vi "Main.vi"() -> ()   [LabVIEW 2018]
uses:
  Initialize/CreateQueue/AllDataQueue.ctl
  Initialize/CreateQueue/SocketQueue.ctl
  Initialize/CreateQueue/LogDataQueue.ctl
  Initialize/CreateQueue/ProDataQueue.ctl
  ProData/SettingData.ctl
  socket/socket.ctl
  Initialize/Setting/DA.ctl
  Initialize/Setting/AD.ctl
  ProData/prodatascan.ctl
  Support/Data.ctl
  <vilib>/DAQmx/read.llb/DAQmx Read (Analog Wfm 1Chan NSamp).vi
  <vilib>/DAQmx/write.llb/DAQmx Write (Analog DBL 1Chan 1Samp).vi
  <vilib>/DAQmx/create/channels.llb/DAQmx Create Channel (AI-Voltage-Basic).vi
  <vilib>/DAQmx/configure/timing.llb/DAQmx Timing (Sample Clock).vi
  <vilib>/DAQmx/miscellaneous.llb/DAQmx Fill In Error Info.vi
  <vilib>/DAQmx/create/channels.llb/DAQmx Create Channel (AO-Voltage-Basic).vi
panel:
  in  "选项卡控件":enum32{"Setting", "Chart"}(tab)
  in  "port":dbl=10003.0
  in  "timeout":i16=-1
  in  "标准差倍数":dbl=5.0
  in  "normal":string="1"
  in  "每通道采样率":u16=60
  in  "电压最大值":u16=5
  in  "电压最小值":i16=-5
  in  "采样率":u16=60000
  in  "接线方式":i32(ring)=10106 items=["默认"=-1, "RSE"=10083, "NRSE"=10078, "差分"=10106, "伪差分"=12529]
  in  "采样模式":i32(ring)=10123 items=["有限采样"=10178, "连续采样"=10123, "硬件定时单点"=12522]
  in  "DA电压最大值":dbl=10.0
  in  "DA电压最小值":dbl=-10.0
  in  "选择通道AD":tag="USB_6211_C34SF/ai1"
  in  "选择通道DA":tag="USB_6211_C34SF/ao1"
  in  "地址":string="8.131.237.84"
  out "选择通道AD  2":tag="USB_6211_2/ai1"
  out "连接状态":string="连接成功"
  in  "adjust":dbl=0.1
  out "波形图表":i32(graph)
  out "nvpai":dbl
  out "max":dbl
  out "min":dbl
  in  "等待时间（毫秒）":u32=20
  out "ADchart":dbl(graph)
  out "DAchart":dbl(graph)
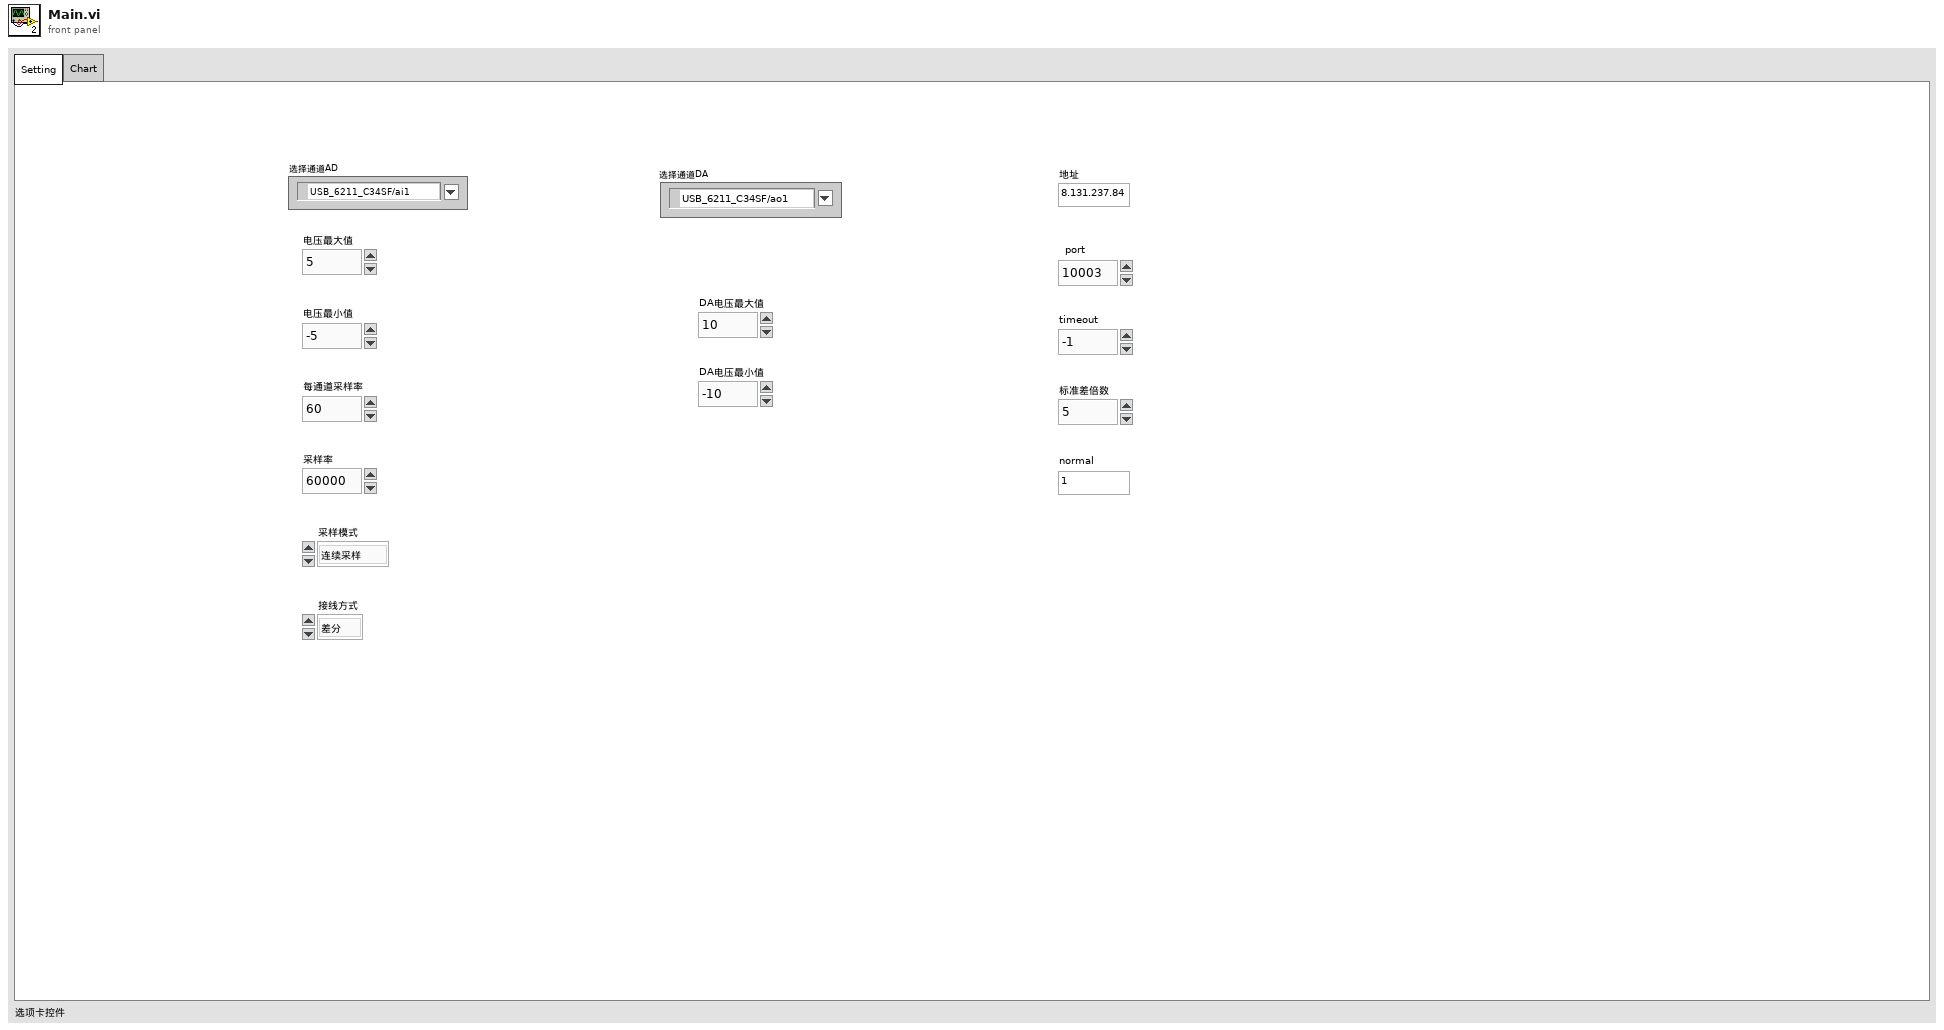
[diagram p1: front panel]
types:
  T1 = typedef "socket.ctl" = cluster{"端口":u16, "timeout":u16, "标准差倍数":dbl, "address":string, "abnormal":string}
  T2 = typedef "DA.ctl" = cluster{"电压最大值":dbl, " 电压最小值":dbl, "选择通道DA ":tag}
  T3 = typedef "AD.ctl" = cluster{"电压最大值":u16, " 电压最小值":i16, " 采样率":u16, "每通道采样率":u16, "采样模式":i32, "接线方式":i32, "source":tag, "选择通道AD ":tag}
  T4 = typedef "Data.ctl" = cluster{"SynQueue":cluster{"SocketQueue":T5, "LogQueue":T6, " DA":refnum<queue>, "ProQueue":T7}, "Error":cluster{"错误输出 2":errorcluster}, "SettingData":T8}
  T5 = typedef "SocketQueue.ctl" = cluster{"ADSTDqueue ":refnum<queue>, "SocketADExceptionqueue":refnum<queue>, "  SocketAD":refnum<queue>}
  T6 = typedef "LogDataQueue.ctl" = cluster{"RunningADqueue":refnum<queue>, "Compensatequeue":refnum<queue>, " RunningDAqueue":refnum<queue>, " RunMin":refnum<queue>}
  T7 = typedef "ProDataQueue.ctl" = cluster{"buffer ":refnum<queue>, " StimeADqueue":refnum<queue>, "  MtimeADqueue":refnum<queue>}
  T8 = typedef "SettingData.ctl" = cluster{"socket":T1, "DA":T2, "AD":T3, "prodatascan":T9}
  T9 = typedef "prodatascan.ctl" = cluster{"max":dbl, "min":dbl, " nvpai":dbl, "初始化数组":dbl[]}
  T10 = typedef "AllDataQueue.ctl" = cluster{"SocketQueue":T5, "LogQueue":T6, " DA":refnum<queue>, "ProQueue":T7}
  T11 = cluster{"max":dbl, "min":dbl, " nvpai":dbl, "初始化数组":dbl[]}
  T12 = cluster{"SocketQueue":T5, "LogQueue":T6, " DA":refnum<queue>, "ProQueue":T7}
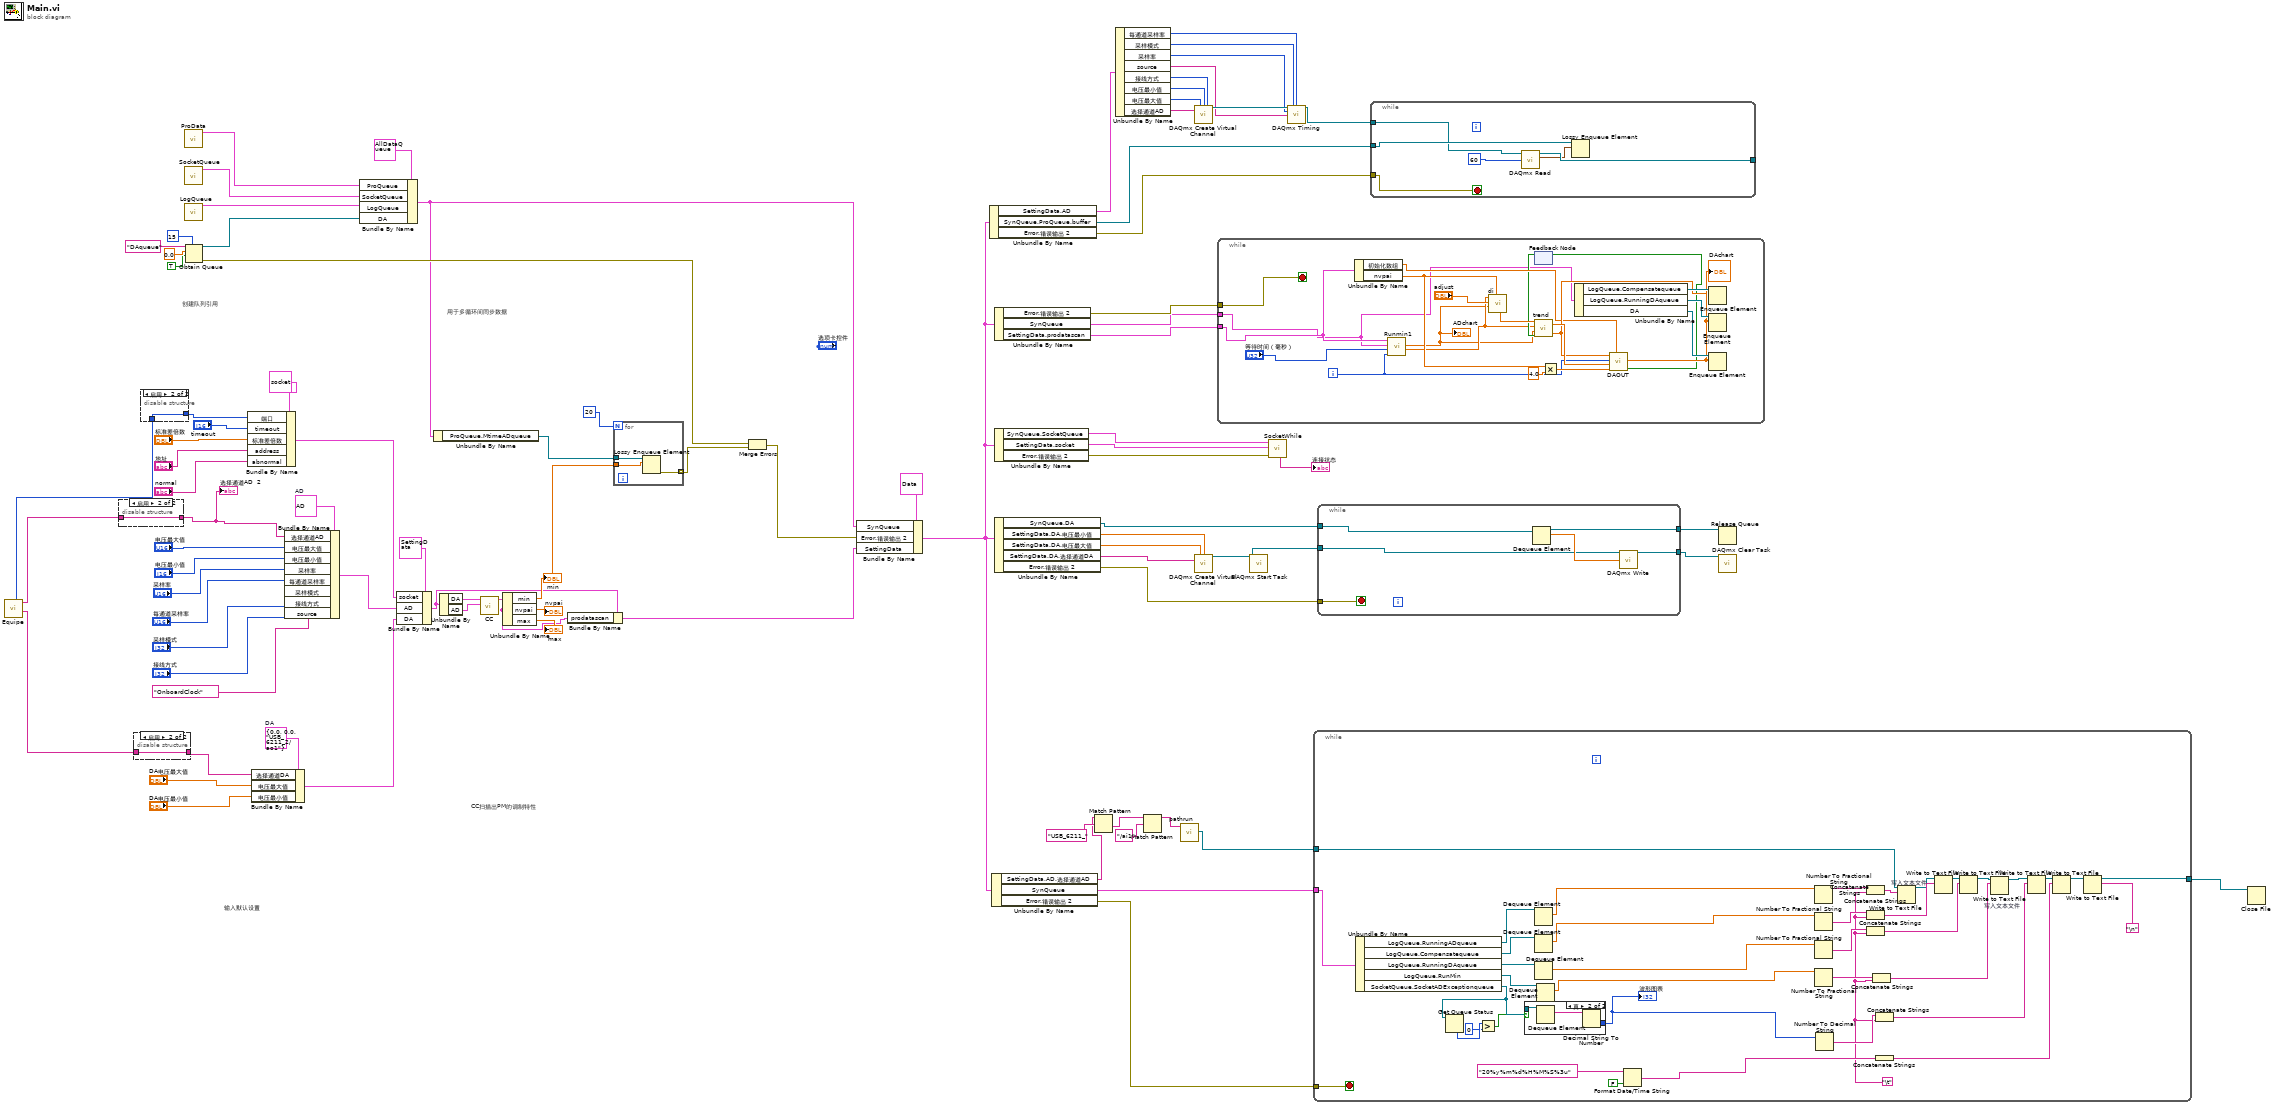
[diagram p0: block diagram]
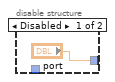
[diagram p2: hidden frame]
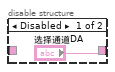
[diagram p3: hidden frame]
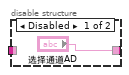
[diagram p4: hidden frame]
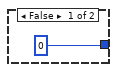
[diagram p5: hidden frame]
diagram:
  w20 = T2 {"电压最大值"=0.0, " 电压最小值"=0.0, "选择通道DA "="USB_6211_2/ao1"}  # DA
  w21 = T3 {"电压最大值"=10013, " 电压最小值"=10013, " 采样率"=10013, "每通道采样率"=10013, "采样模式"=10123, "接线方式"=10106, "source"="OnboardClock", "选择通道AD "="USB_6211_2/ai1"}  # AD
  # "CC扫描出PM的调制特性"
  # "输入默认设置"
  # "用于多循环间同步数据"
  # "创建队列引用"
  n1 = call "Equipe.vi"() -> ("DA"=w4:string, "AD"=w5:string, "port"=w3:i32)  [unwired: 8 in, 1 out]
  n2 = disable-structure shown="启用" {
    disable-tunnel: ["选择通道AD" w91] -> w6
    disable-tunnel: w5 -> [_ w91]
    frame Disabled {
    }
    frame Enabled {
    }
  }
  "选择通道AD  2" <- w6
  n3 = disable-structure shown="启用" {
    disable-tunnel: ["选择通道DA" w93] -> w67
    disable-tunnel: w4 -> [_ w93]
    frame Disabled {
    }
    frame Enabled {
    }
  }
  n4 = disable-structure shown="启用" {
    disable-tunnel: ["port" w95] -> w1
    disable-tunnel: w3 -> [_ w95]
    frame Disabled {
    }
    frame Enabled {
    }
  }
  n5 = call "ProData.vi"() -> ("ProDataQueue"=w81:T7)  [unwired: 11 in]
  n6 = call "SocketQueue.vi"() -> ("SocketQueue"=w83:T5)  [unwired: 11 in]
  n7 = call "LogQueue.vi"() -> ("LogQueue"=w82:T6)  [unwired: 11 in]
  n8 = Obtain Queue(max queue size (-1, unlimited)=15 ("队列最大值（-1，无限）"), name (unnamed)="DAqueue" ("名称（未命名）"), element data type=0.0, create if not found? (T)=TRUE ("如未找到则创建？(T)")) -> (queue out=w84:refnum<queue>, error out=w60:errorcluster)  [unwired: 1 in, 1 out]
  n9 = Bundle By Name(cluster=T1 {"端口"=10013, "timeout"=10013, "标准差倍数"=0.0, "address"="{\"ad\":1}", "abnormal"="{\"ad\":0}"} ("socket"), "端口"=w1, "timeout"="timeout", "标准差倍数"="标准差倍数", "address"="地址", "abnormal"="normal") -> (w71:T1)
  n10 = Bundle By Name(cluster=w20, "选择通道DA"=w67, "电压最大值"="DA电压最大值", "电压最小值"="DA电压最小值") -> (w66:T2)
  n11 = Bundle By Name(cluster=w21, "选择通道AD"=w6, "电压最大值"="电压最大值", "电压最小值"="电压最小值", "采样率"="采样率", "每通道采样率"="每通道采样率", "采样模式"="采样模式", "接线方式"="接线方式", "source"=tag "OnboardClock") -> (w65:T3)
  n12 = Bundle By Name(cluster=T10 {"SocketQueue"={"ADSTDqueue "=refnum, "SocketADExceptionqueue"=refnum, "  SocketAD"=refnum}, "LogQueue"={"RunningADqueue"=refnum, "Compensatequeue"=refnum, " RunningDAqueue"=refnum, " RunMin"=refnum}, " DA"=refnum, "ProQueue"={"buffer "=refnum, " StimeADqueue"=refnum, "  MtimeADqueue"=refnum}}, "ProQueue"=w81, "SocketQueue"=w83, "LogQueue"=w82, "DA"=w84) -> (w50:T10)
  n13 = Bundle By Name(cluster=T8 {"socket"={"端口"=10013, "timeout"=10013, "标准差倍数"=0.0, "address"="{\"ad\":1}", "abnormal"="{\"ad\":0}"}, "DA"={"电压最大值"=0.0, " 电压最小值"=0.0, "选择通道DA "="USB_6211_2/ao1"}, "AD"={"电压最大值"=10013, " 电压最小值"=10013, " 采样率"=10013, "每通道采样率"=10013, "采样模式"=10123, "接线方式"=10106, "source"="OnboardClock", "选择通道AD "="USB_6211_2/ai1"}, "prodatascan"={"max"=0.0, "min"=0.0, " nvpai"=0.0, "初始化数组"=[]}} ("SettingData"), "socket"=w71, "AD"=w65, "DA"=w66) -> (w10:T8)
  n14 = Unbundle By Name(w50) -> ("ProQueue.MtimeADqueue"=w62:refnum<queue>)
  n15 = Unbundle By Name(w10) -> ("DA"=w63:T2, "AD"=w64:T3)
  n16 = call "CC.vi"("AD"=w64, "DA"=w63) -> ("prodatascan"=w9:T11)  [unwired: 8 in, 1 out]
  n17 = Unbundle By Name(w9) -> ("min"=w13:dbl, "nvpai"=→"nvpai":dbl, "max"=→"max":dbl)
  "min" <- w13
  n18 = Bundle By Name(cluster=w10, "prodatascan"=w9) -> (w8:T8)
  n19 = for {
    N: 20 -> [_]
    tunnel: w62 -> [w98]
    tunnel: w13 -> [w97]
    tunnel: [w96] -> w59 mode=indexing
    n20 = Lossy Enqueue Element(queue=w98, element=w97) -> (error out=w96:errorcluster)  [unwired: 1 in, 3 out]
  }
  n21 = Merge Errors(w60, w59) -> (w40:errorcluster)
  n22 = Bundle By Name(cluster=T4 {"SynQueue"={"SocketQueue"={"ADSTDqueue "=refnum, "SocketADExceptionqueue"=refnum, "  SocketAD"=refnum}, "LogQueue"={"RunningADqueue"=refnum, "Compensatequeue"=refnum, " RunningDAqueue"=refnum, " RunMin"=refnum}, " DA"=refnum, "ProQueue"={"buffer "=refnum, " StimeADqueue"=refnum, "  MtimeADqueue"=refnum}}, "Error"={"错误输出 2"={"status"=FALSE, "code"=0, "source"=""}}, "SettingData"={"socket"={"端口"=0, "timeout"=0, "标准差倍数"=0.0, "address"="{\"ad\":1}", "abnormal"="{\"ad\":0}"}, "DA"={"电压最大值"=0.0, " 电压最小值"=0.0, "选择通道DA "="USB_6211_2/ao1"}, "AD"={"电压最大值"=10013, " 电压最小值"=10013, " 采样率"=10013, "每通道采样率"=10013, "采样模式"=10123, "接线方式"=10106, "source"="OnboardClock", "选择通道AD "="USB_6211_2/ai1"}, "prodatascan"={"max"=0.0, "min"=0.0, " nvpai"=0.0, "初始化数组"=[]}}}, "SynQueue"=w50, "Error.错误输出 2"=w40, "SettingData"=w8) -> (w25:T4)
  n23 = Unbundle By Name(w25) -> ("SettingData.AD"=w28:T3, "SynQueue.ProQueue.buffer"=w38:refnum<queue>, "Error.错误输出 2"=w39:errorcluster)
  n24 = Unbundle By Name(w25) -> ("SettingData.AD.选择通道AD"=w7:tag, "SynQueue"=w24:T12, "Error.错误输出 2"=w23:errorcluster)
  n25 = Unbundle By Name(w25) -> ("Error.错误输出 2"=w53:errorcluster, "SynQueue"=w51:T12, "SettingData.prodatascan"=w52:T9)
  n26 = Unbundle By Name(w25) -> ("SynQueue.SocketQueue"=w54:T5, "SettingData.socket"=w15:T1, "Error.错误输出 2"=w55:errorcluster)
  n27 = Unbundle By Name(w25) -> ("SynQueue.DA"=w44:refnum<queue>, "SettingData.DA.电压最小值"=w47:dbl, "SettingData.DA.电压最大值"=w43:dbl, "SettingData.DA.选择通道DA"=w48:tag, "Error.错误输出 2"=w49:errorcluster)
  n28 = Match Pattern(string=w7, regular expression="USB_6211_" ("正则表达式")) -> (after substring=w18:string)  [unwired: 1 in, 3 out]
  n29 = Unbundle By Name(w28) -> ("每通道采样率"=w29:u16, "采样模式"=w30:i32, "采样率"=w31:u16, "source"=w32:tag, "接线方式"=w37:i32, "电压最小值"=w36:i16, "电压最大值"=w35:u16, "选择通道AD"=w34:tag)
  n30 = Match Pattern(string=w18, regular expression="/ai1" ("正则表达式")) -> (before substring=w16:string)  [unwired: 1 in, 3 out]
  n31 = call "pathrun.vi"("时间格式字符串(%c)"=w16) -> ("引用句柄输出"=w26:refnum<file>)  [unwired: 10 in]
  n32 = call-poly <vilib>:"DAQmx Create Virtual Channel.vi"("maximum value"=w35, "minimum value"=w36, "input terminal configuration"=w37, "physical channels"=w34) -> ("task out"=w33:refnum<k21>)  [unwired: 10 in, 1 out]
  n33 = call-poly <vilib>:"DAQmx Create Virtual Channel.vi"("maximum value"=w43, "minimum value"=w47, "physical channels"=w48) -> ("task out"=w46:refnum<k21>)  [unwired: 11 in, 1 out]
  n34 = while {
    tunnel: w53 -> [w117]
    tunnel: w51 -> [w101]
    tunnel: w52 -> [w102]
    i -> [w100]
    stop <- w117 stop-if-true
    n35 = Unbundle By Name(w102) -> ("初始化数组"=w108:dbl[], "nvpai"=w105:dbl)
    n36 = call "Runmin1.vi"("循环次数 i"=w100, "等待时间（毫秒）"="等待时间（毫秒）", "Queue1"=w101, "prodatascan"=w102) -> ("runMin"=w104:dbl, "AD"=w103:dbl)  [unwired: 6 in]
    "ADchart" <- w103
    n37 = call "di.vi"("RunMin"=w104, "adjust"="adjust", "AD"=w103, "Nvpai"=w105) -> ("Compensate1"=w118:dbl)  [unwired: 6 in]
    n38 = feedback #1() -> (w106:bool)  [unwired: 1 in]
    n39 = call "trend.vi"("jumpBool"=w106, "AD"=w103, "runMin"=w104, "Compensate1"=w118) -> ("Compensate1Out"=w109:dbl, "changeSymbol"=w110:dbl)
    n40 = Multiply(x=w105, y=4.0) -> (x*y=w111:dbl)
    n41 = Unbundle By Name(w101) -> ("LogQueue.Compensatequeue"=w116:refnum<queue>, "LogQueue.RunningDAqueue"=w115:refnum<queue>, "DA"=w113:refnum<queue>)
    n42 = call "DAOUT.vi"("maxInitial数组"=w108, "maxInitialVoltage"=w111, "changeSymbol"=w110, "running recycle counter"=w100, "compensate"=w109) -> ("jump symbol"=w107:bool, "real running DA output"=w112:dbl)  [unwired: 5 in]
    "DAchart" <- w112
    n43 = feedback-in #1(w107) -> ()
    n44 = Enqueue Element(queue=w116, element=w109) -> ()  [unwired: 2 in, 3 out]
    n45 = Enqueue Element(queue=w115, element=w112) -> ()  [unwired: 2 in, 3 out]
    n46 = Enqueue Element(queue=w113, element=w112) -> ()  [unwired: 2 in, 3 out]
  }
  n47 = call <vilib>:"DAQmx Start Task.vi"("task/channels in"=w46) -> ("task out"=w45:refnum<k21>)  [unwired: 13 in, 1 out]
  n48 = call "SocketWhile.vi"("error out"=w55, "socket 2"=w15, "SocketQueue"=w54) -> ("socket"=→"连接状态":string)  [unwired: 8 in]
  n49 = call-poly <vilib>:"DAQmx Timing.vi"("task/channels in"=w33, "sample mode"=w30, "samples per channel"=w29, "rate"=w31, "source"=w32) -> ("task out"=w27:refnum<k21>)  [unwired: 9 in, 1 out]
  n50 = while {
    tunnel: w23 -> [w153]
    tunnel: [w123] -> w22
    tunnel: w26 -> [w122]
    tunnel: w24 -> [w120]
    stop <- w153 stop-if-true
    w121 = "\t"
    n51 = Unbundle By Name(w120) -> ("LogQueue.RunningADqueue"=w152:refnum<queue>, "LogQueue.Compensatequeue"=w156:refnum<queue>, "LogQueue.RunningDAqueue"=w155:refnum<queue>, "LogQueue.RunMin"=w154:refnum<queue>, "SocketQueue.SocketADExceptionqueue"=w151:refnum<queue>)
    n52 = Get Queue Status(queue=w151) -> (# elements in queue=w150:i32)  [unwired: 2 in, 7 out]
    n53 = Greater?(x=w150, y=0) -> (0:w148:bool)
    n54 = case shown="真" w148 {
      tunnel: [0 w161] -> w128
      tunnel: w151 -> [_ w160]
      frame False {
      }
      frame True {
        n55 = Dequeue Element(queue=w160) -> (element=w162:string)  [unwired: 2 in, 3 out]
        n56 = Decimal String To Number(string=w162) -> (number=w161:i32)  [unwired: 2 in, 1 out]
      }
    }
    "波形图表" <- w128
    n57 = Dequeue Element(queue=w152) -> (element=w138:dbl)  [unwired: 2 in, 3 out]
    n58 = Dequeue Element(queue=w156) -> (element=w137:dbl)  [unwired: 2 in, 3 out]
    n59 = Dequeue Element(queue=w155) -> (element=w136:dbl)  [unwired: 2 in, 3 out]
    n60 = Dequeue Element(queue=w154) -> (element=w130:dbl)  [unwired: 2 in, 3 out]
    n61 = Format Date/Time String(time format string (%c)="20%y%m%d%H%M%S%3u" ("时间格式字符串(%c)"), UTC format=FALSE ("UTC格式")) -> (date/time string=w126:string)  [unwired: 1 in]
    n62 = Number To Fractional String(number=w138) -> (F-format string=w143:string)  [unwired: 3 in]
    n63 = Number To Fractional String(number=w137) -> (F-format string=w145:string)  [unwired: 3 in]
    n64 = Number To Fractional String(number=w136) -> (F-format string=w146:string)  [unwired: 3 in]
    n65 = Number To Fractional String(number=w130) -> (F-format string=w131:string)  [unwired: 3 in]
    n66 = Number To Decimal String(number=w128) -> (decimal integer string=w127:string)  [unwired: 1 in]
    n67 = Concatenate Strings(w143, w121) -> (w140:string)
    n68 = Concatenate Strings(w145, w121) -> (w142:string)
    n69 = Concatenate Strings(w146, w121) -> (w147:string)
    n70 = Concatenate Strings(w131, w121) -> (w129:string)
    n71 = Concatenate Strings(w127, w121) -> (w125:string)
    n72 = Concatenate Strings(w126) -> (w124:string)
    n73 = Write to Text File "写入文本文件"(file (use dialog)=w122, text=w140) -> (refnum out=w141:refnum<file>)  [unwired: 2 in, 2 out]
    n74 = Write to Text File(file (use dialog)=w141, text=w142) -> (refnum out=w144:refnum<file>)  [unwired: 2 in, 2 out]
    n75 = Write to Text File(file (use dialog)=w144, text=w147) -> (refnum out=w133:refnum<file>)  [unwired: 2 in, 2 out]
    n76 = Write to Text File "写入文本文件"(file (use dialog)=w133, text=w129) -> (refnum out=w134:refnum<file>)  [unwired: 2 in, 2 out]
    n77 = Write to Text File(file (use dialog)=w134, text=w125) -> (refnum out=w135:refnum<file>)  [unwired: 2 in, 2 out]
    n78 = Write to Text File(file (use dialog)=w135, text=w124) -> (refnum out=w132:refnum<file>)  [unwired: 2 in, 2 out]
    n79 = Write to Text File(file (use dialog)=w132, text="\n") -> (refnum out=w123:refnum<file>)  [unwired: 2 in, 2 out]
  }
  n80 = while {
    tunnel: [w168] -> w41
    tunnel: [w167] -> w42
    tunnel: w44 -> [w164]
    tunnel: w49 -> [w165]
    tunnel: w45 -> [w163]
    stop <- w165 stop-if-true
    n81 = Dequeue Element(queue=w164) -> (queue out=w167:refnum<queue>, element=w166:dbl)  [unwired: 2 in, 2 out]
    n82 = call-poly <vilib>:"DAQmx Write.vi"("task/channels in"=w163, "data"=w166) -> ("task out"=w168:refnum<k21>)  [unwired: 11 in, 2 out]
  }
  n83 = while {
    tunnel: [w174] -> _
    tunnel: w38 -> [w171]
    tunnel: w39 -> [w170]
    tunnel: w27 -> [w169]
    stop <- w170 stop-if-true
    n84 = call-poly <vilib>:"DAQmx Read.vi"("task/channels in"=w169, "number of samples per channel"=60) -> ("task out"=w174:refnum<k21>, "data"=w173:waveform(dbl))  [unwired: 11 in, 1 out]
    n85 = Lossy Enqueue Element(queue=w171, element=w173) -> ()  [unwired: 1 in, 4 out]
  }
  n86 = Release Queue(queue=w42) -> ()  [unwired: 2 in, 3 out]
  n87 = call <vilib>:"DAQmx Clear Task.vi"("task in"=w41) -> ()  [unwired: 14 in, 1 out]
  n88 = Close File(refnum=w22) -> ()  [unwired: 1 in, 2 out]
